vi "Read timeout.vi"(11 "Network Endpoint in":refnum<class "Network Endpoint.lvclass">) -> (2 "timeout":i32 min=0 max=5000)   [LabVIEW 2020, in "Network Endpoint.lvlib" / "Network Endpoint.lvclass"]
doc: "Returns the timeout specified for this endpoint. This timeout limits both the time to wait for a connection and the time to wait for messages from the remote endpoint once a connection has been established."
uses:
  Network Endpoint.lvclass
  Network Endpoint.lvclass/Network Endpoint.ctl
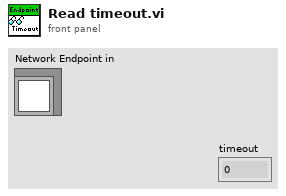
[diagram p1: front panel]
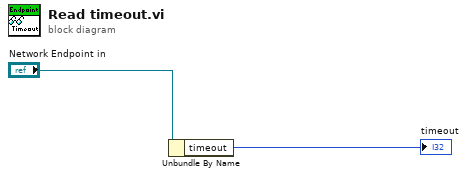
[diagram p0: block diagram]
diagram:
  n1 = Unbundle By Name("Network Endpoint in") -> ("timeout"=→"timeout":i32)
